vi "AG Elapsed Time.vi"(5 "Auto Reset (F)":bool caption="Auto Reset", 6 "precision (3)":i16=3, 7 "Reset":bool, 8 "error in (no error)":errorcluster, 10 "Time Target (10s)":dbl=1.0 caption="Time Target (s)") -> (0 "error out":errorcluster, 2 "Time has Elapsed":bool, 3 "Elapsed Time":dbl)   [LabVIEW 2012]
doc: "A simple wrapper around the elapsed time function that adds formating for common display cases."
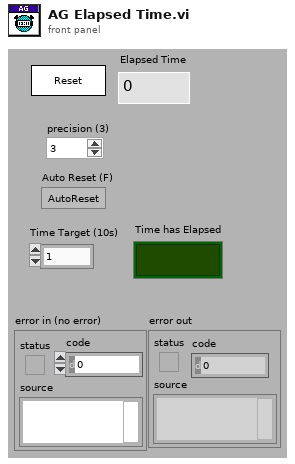
[diagram p1: front panel]
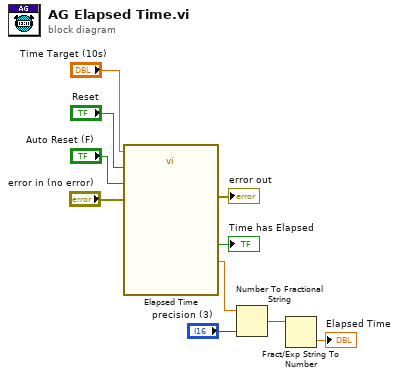
[diagram p0: block diagram]
diagram:
  n1 = call "Elapsed Time"("Time Target (s)"="Time Target (10s)", "Reset"="Reset", "Auto Reset"="Auto Reset (F)", "error in (no error)"="error in (no error)") -> ("Elapsed Time (s)"=w7:dbl, "Time has Elapsed"=→"Time has Elapsed":bool, "error out"=→"error out":errorcluster)  [unwired: 8 in, 5 out]
  n2 = Number To Fractional String(number=w7, precision (6)="precision (3)") -> (F-format string=w10:string)  [unwired: 2 in]
  n3 = Fract/Exp String To Number(string=w10) -> (number=→"Elapsed Time":dbl)  [unwired: 3 in, 1 out]
